vi "Array-Intersection.vi"(10 "B":dbl[](array[numeric]), 11 "A":dbl[](array[numeric])) -> (0 "intersection":dbl[](array[numeric]), 2 "iB":i32[](array[numeric]), 3 "iA":i32[](array[numeric]))   [LabVIEW 2020]
uses:
  Comparison VIs/Approx Equal (1D-Scalar).vi
  <vilib>/Analysis/polynomials.llb/Unique Numbers and Multiplicity (DBL).vi
  <vilib>/Analysis/NI_AALPro.lvlib
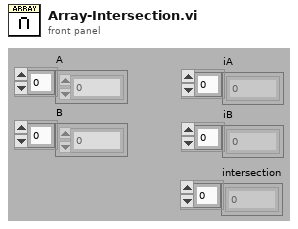
[diagram p1: front panel]
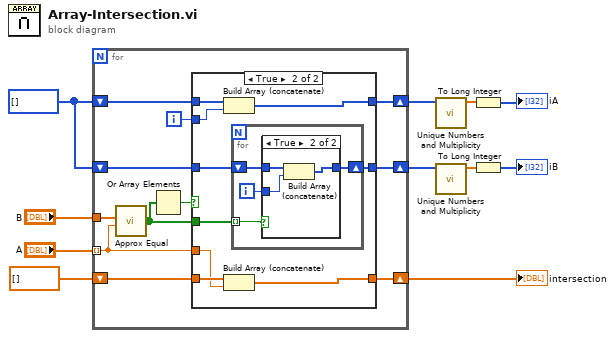
[diagram p0: block diagram]
diagram:
  w8 = i32[] [] ("iA")
  n1 = for {
    tunnel: "A" -> [w13] mode=indexing
    tunnel: "B" -> [w12]
    shift-right: [w18] -> w7
    shift-left: dbl[] [] ("intersection") -> [w19]
    shift-right: [w17] -> w3
    shift-left: w8 -> [w20]
    shift-right: [w15] -> w6
    shift-left: w8 -> [w16]
    i -> [w14]
    n2 = call-poly "Approx Equal.vi"("Y"=w13, "X"=w12) -> ("X approx Y?"=w21:bool[])  [unwired: 4 in]
    n3 = Or Array Elements(Boolean array=w21) -> (logical OR=w22:bool)
    n4 = case shown="True" w22 {
      tunnel: w21 -> [_ w26]
      tunnel: w20 -> [w24 w34]
      tunnel: w19 -> [w25 w32]
      tunnel: [w25 w29] -> w18
      tunnel: [w24 w31] -> w17
      tunnel: w16 -> [w23 w33]
      tunnel: [w23 w27] -> w15
      tunnel: w14 -> [_ w30]
      tunnel: w13 -> [_ w28]
      frame False {
      }
      frame True {
        n5 = Build Array (concatenate)(w34, w30) -> (w31:i32[])
        n6 = Build Array (concatenate)(w32, w28) -> (w29:dbl[])
        n7 = for {
          shift-right: [w37] -> w27
          shift-left: w33 -> [w38]
          tunnel: w26 -> [w36] mode=indexing
          i -> [w35]
          n8 = case shown="True" w36 {
            tunnel: w38 -> [w39 w42]
            tunnel: [w39 w41] -> w37
            tunnel: w35 -> [_ w40]
            frame False {
            }
            frame True {
              n9 = Build Array (concatenate)(w42, w40) -> (w41:i32[])
            }
          }
        }
      }
    }
  }
  "intersection" <- w7
  n10 = call-poly <vilib>:"Unique Numbers and Multiplicity.vi"("Numbers"=w3) -> ("Unique Numbers"=w2:dbl[])  [unwired: 8 in, 2 out]
  n11 = call-poly <vilib>:"Unique Numbers and Multiplicity.vi"("Numbers"=w6) -> ("Unique Numbers"=w5:dbl[])  [unwired: 8 in, 2 out]
  n12 = To Long Integer(number=w2) -> (32bit integer=→"iA":i32[])
  n13 = To Long Integer(number=w5) -> (32bit integer=→"iB":i32[])
